vi "GetFirstScreen.vi"(8 "error in (no error)":errorcluster, 11 "Menu in":refnum<class "Menu.lvclass">) -> (0 "error out":errorcluster, 2 "Array":u32[][](array[numeric]), 3 "Menu out":refnum<class "Menu.lvclass">)   [LabVIEW 2019, in "RT_Game.lvlib" / "Menu.lvclass"]
uses:
  Menu.lvclass
  Game/Game.lvclass
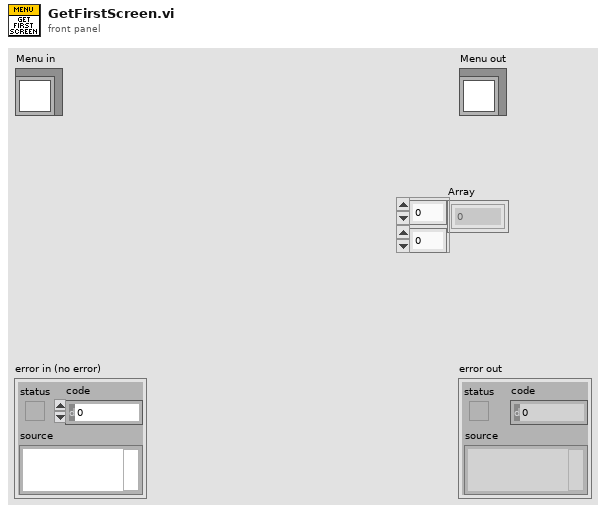
[diagram p1: front panel]
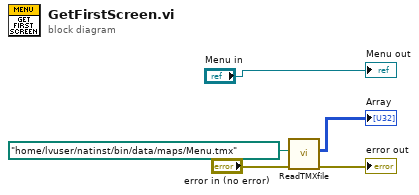
[diagram p0: block diagram]
diagram:
  n1 = call "ReadTMXfile.vi"("error in (no error)"="error in (no error)", "path to tmx-file (created with Tiles2D)"=path "/home/lvuser/natinst/bin/data/maps/Menu.tmx") -> ("error out"=→"error out":errorcluster, "Tilenumbers"=→"Array":u32[][])  [unwired: 8 in]
  "Menu out" <- "Menu in"
